vi "Default controls - save controls values.vi"(8 "error in (no error)":errorcluster) -> (0 "error out":errorcluster)   [LabVIEW 2020]
uses:
  Save-Load-Defaults.lvlib/Save-Load-Defaults.lvlib
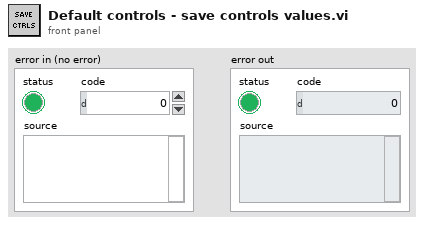
[diagram p1: front panel]
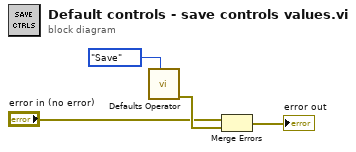
[diagram p0: block diagram]
diagram:
  n1 = call "Defaults Operator.vi"("Operation (Load)"=enum16{"Load", "Save"}."Save") -> ("error out"=w3:errorcluster)  [unwired: 8 in, 2 out]
  n2 = Merge Errors("error in (no error)", w3) -> (→"error out":errorcluster)
